vi "Eliminate Deadband.vi"(11 "Motor In":dbl) -> (3 "Scaled Motor":dbl)   [LabVIEW 2013]
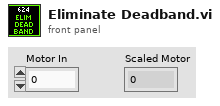
[diagram p1: front panel]
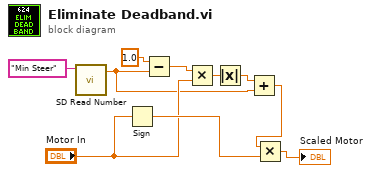
[diagram p0: block diagram]
diagram:
  n1 = call <vilib>:"SD Read Number.vi"("Name"="Min Steer") -> ("Numeric"=w6:dbl)  [unwired: 8 in, 2 out]
  n2 = Sign(1:"Motor In") -> (0:w10:dbl)
  n3 = Subtract(x=1.0, y=w6) -> (x-y=w3:dbl)
  n4 = Multiply(x=w3, y="Motor In") -> (x*y=w4:dbl)
  n5 = Absolute Value(x=w4) -> (abs(x)=w5:dbl)
  n6 = Add(x=w5, y=w6) -> (x+y=w9:dbl)
  n7 = Multiply(x=w9, y=w10) -> (x*y=→"Scaled Motor":dbl)
